vi "LimitDataAccess.vi"() -> ()   [LabVIEW 2019]
uses:
  <vilib>/addons/database/Connection.llb/DB Tools Open Connec (String).vi
  <vilib>/addons/database/NI_Database_API.lvlib
panel:
  in  "Connection Information":string
  out "Limited Data Access":variant[][](array[variant])
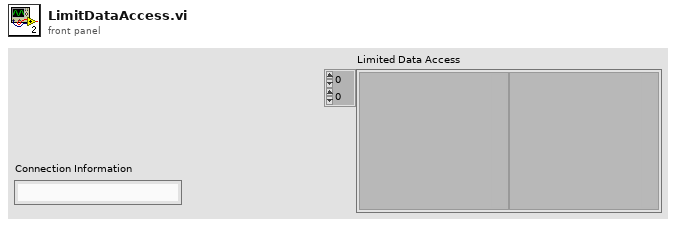
[diagram p1: front panel]
types:
  T1 = typedef "NI_Database_API.lvlib/Conn ObjectReference.ctl" = refnum<k1>
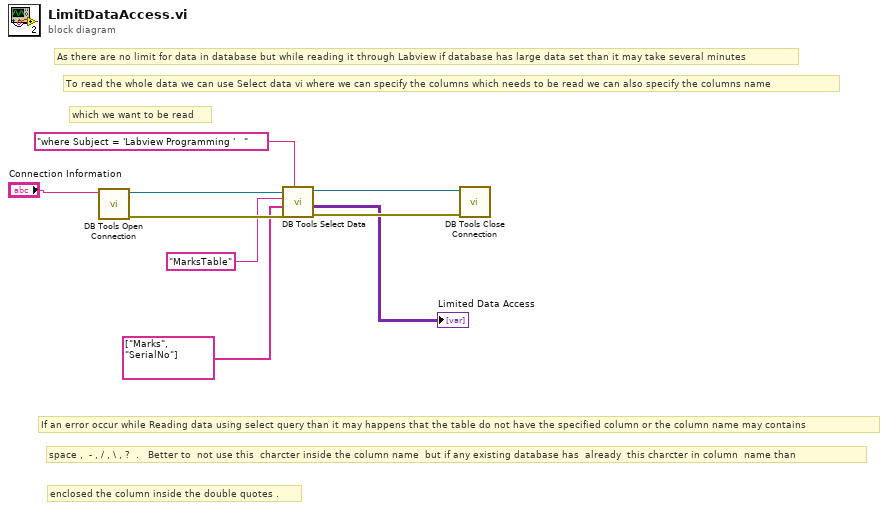
[diagram p0: block diagram]
diagram:
  # "enclosed the column inside the double quotes ."
  # "space ,  - , / , \\ , ?  .   Better to  not use this  charcter inside the column name  but if any existing database has  already  this charcter in column  name than"
  # "If an error occur while Reading data using select query than it may happens that the table do not have the specified column or the column name may contains"
  # "which we want to be read"
  # "To read the whole data we can use Select data vi where we can specify the columns which needs to be read we can also specify the columns name"
  # "As there are no limit for data in database but while reading it through Labview if database has large data set than it may take several minutes"
  n1 = call-poly <vilib>:"DB Tools Open Connection.vi"("connection information"="Connection Information") -> ("error out"=w8:errorcluster, "connection reference"=w9:T1)  [unwired: 7 in]
  n2 = call <vilib>:"DB Tools Select Data.vi"("condition"="where Subject = 'Labview Programming '   ", "error in (no error)"=w8, "columns"=string[] ["Marks", "SerialNo"], "table"="MarksTable", "connection reference"=w9) -> ("error out"=w6:errorcluster, "data"=→"Limited Data Access":variant[][], "connection reference out"=w7:T1)  [unwired: 1 in]
  n3 = call <vilib>:"DB Tools Close Connection.vi"("error in (no error)"=w6, "connection reference"=w7) -> ()  [unwired: 5 in, 1 out]
